vi "Is DAA.vi"(8 "error in (no error)":errorcluster, 11 "Model in":refnum<class "Model.lvclass">) -> (0 "error out":errorcluster, 2 "IsDAA":bool, 3 "Model out":refnum<class "Model.lvclass">)   [LabVIEW 2016]
uses:
  Common_RT_FAILC/DataTypes/HPTypes.ctl
  Common_RT_FAILC/RTHPILC.lvlib
  Model.lvclass
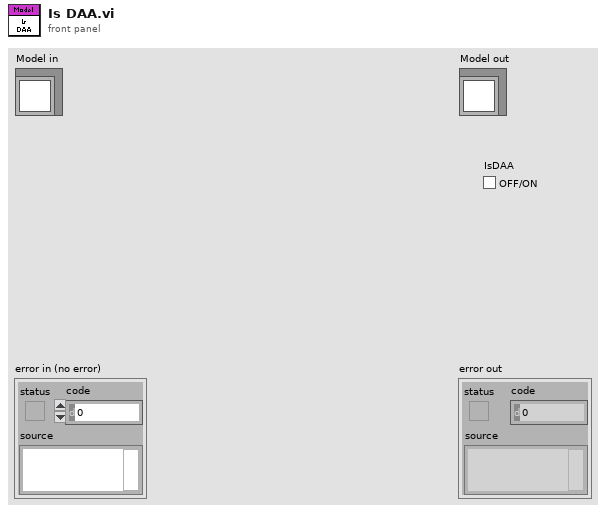
[diagram p1: front panel]
types:
  T1 = typedef "RTHPILC.lvlib/HPTypes.ctl" = enum16{"SingleAxis", "LateralDualAxis", "CrossLateralDualAxis"}
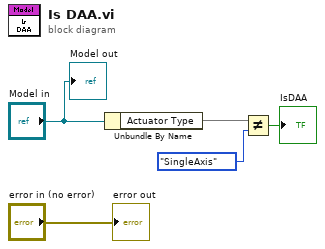
[diagram p0: block diagram]
diagram:
  n1 = Unbundle By Name("Model in") -> ("Actuator Type"=w5)
  n2 = Not Equal?(x=w5, y=HPTypes."SingleAxis") -> (x != y?=→"IsDAA":bool)
  "error out" <- "error in (no error)"
  "Model out" <- "Model in"
